vi "test.vi"() -> ()   [LabVIEW 2021]
uses:
  IChair/CushionModel.ctl
  ITable/TableclothType.ctl
  Chair/Chair.lvclass
  IChair/IChair.lvclass
  Table/Table.lvclass
  ITable/ITable.lvclass
panel:
  out "Cusioon  test Results":string[](array[string])
  out "Setup Result":string[](array[string])
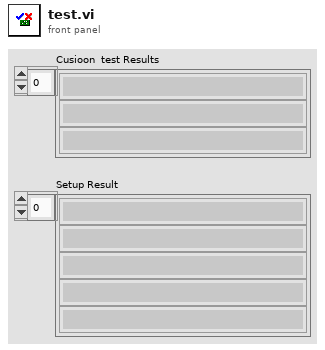
[diagram p1: front panel]
types:
  T1 = typedef "ITable.lvclass/TableclothType.ctl" = u16
  T2 = typedef "IChair.lvclass/CushionModel.ctl" = u16
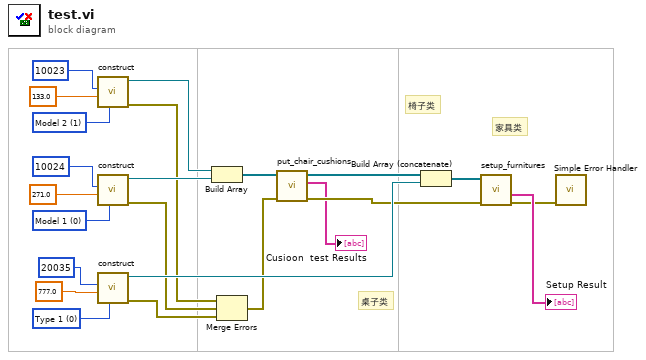
[diagram p0: block diagram]
diagram:
  w13 = T1 0 items=["Type 1", "Type 2"] ("tablecloth_type")
  w18 = T2 1 items=["Model 1", "Model 2"] ("cushion_model")
  w19 = T2 0 items=["Model 1", "Model 2"] ("cushion_model")
  # "家具类"
  # "椅子类"
  # "桌子类"
  n1 = call "construct.vi"("cushion_model"=w18, "cost"=133.0 ("price"), "id"=u32 10023) -> ("error out"=w6:errorcluster, "Chair out"=w11:refnum<class "Chair.lvclass">)  [unwired: 7 in]
  n2 = call "construct.vi"("cushion_model"=w19, "cost"=271.0 ("price"), "id"=u32 10024) -> ("error out"=w5:errorcluster, "Chair out"=w10:refnum<class "Chair.lvclass">)  [unwired: 7 in]
  n3 = call "construct.vi"("tablecloth_type"=w13, "cost"=777.0 ("price"), "id"=u32 20035) -> ("error out"=w4:errorcluster, "table out"=w12:refnum<class "Table.lvclass">)  [unwired: 7 in]
  n4 = Build Array "Build Array"(w11, w10) -> (w9:refnum<class "Chair.lvclass">[])
  n5 = Merge Errors(w6, w5, w4) -> (w3:errorcluster)
  n6 = call "put_chair_cushions.vi"("error in"=w3, "chairs in"=w9) -> ("error out"=w7:errorcluster, "cushion results"=→"Cusioon  test Results":string[], "chairs out"=w8:refnum<class "IChair.lvclass">[])  [unwired: 7 in]
  n7 = Build Array (concatenate) "Build Array"(w8, w12) -> (w17:refnum<class "IFurniture.lvclass">[])
  n8 = call "setup_furnitures.vi"("error in"=w7, "furntures in"=w17) -> ("error out"=w1:errorcluster, "setup results"=→"Setup Result":string[])  [unwired: 7 in, 1 out]
  n9 = call <vilib>:"Simple Error Handler.vi"("error in (no error)"=w1) -> ()  [unwired: 4 in, 5 out]
